vi "CheckI16_Range.vi"(8 "Step":i16, 11 "Current":i16) -> (3 "In Range Value":i16)   [LabVIEW 2016]
panel:
  # "Copyright (C) 2020 Edward S Allgeyer\n\nRedistribution and use in source and binary forms, with or without\nmodification, are permitted provided that the following conditions\nare met:\n\n1. Redistributions of source code must retain the above copyright\n   notice, this list of conditions and the following disclaimer.\n\n2. Redistributions in binary form must reproduce the above copyright\n   notice, this list of conditions and the following disclaimer in\n   the documentation and/or other materials provided with the\n   distribution.\n\n3. Neither the name of the copyright holder nor the names of its\n   contributors may be used to endorse or promote products derived\n   from this software without specific prior written permission.\n\nTHIS SOFTWARE IS PROVIDED BY THE COPYRIGHT HOLDERS AND CONTRIBUTORS\n\"AS IS\" AND ANY EXPRESS OR IMPLIED WARRANTIES, INCLUDING, BUT NOT\nLIMITED TO, THE IMPLIED WARRANTIES OF MERCHANTABILITY AND FITNESS\nFOR A PARTICULAR PURPOSE ARE DISCLAIMED. IN NO EVENT SHALL THE\nCOPYRIGHT HOLDER OR CONTRIBUTORS BE LIABLE FOR ANY DIRECT, INDIRECT,\nINCIDENTAL, SPECIAL, EXEMPLARY, OR CONSEQUENTIAL DAMAGES (INCLUDING,\nBUT NOT LIMITED TO, PROCUREMENT OF SUBSTITUTE GOODS OR SERVICES;\nLOSS OF USE, DATA, OR PROFITS; OR BUSINESS INTERRUPTION) HOWEVER\nCAUSED AND ON ANY THEORY OF LIABILITY, WHETHER IN CONTRACT, STRICT\nLIABILITY, OR TORT (INCLUDING NEGLIGENCE OR OTHERWISE) ARISING IN\nANY WAY OUT OF THE USE OF THIS SOFTWARE, EVEN IF ADVISED OF THE\nPOSSIBILITY OF SUCH DAMAGE."
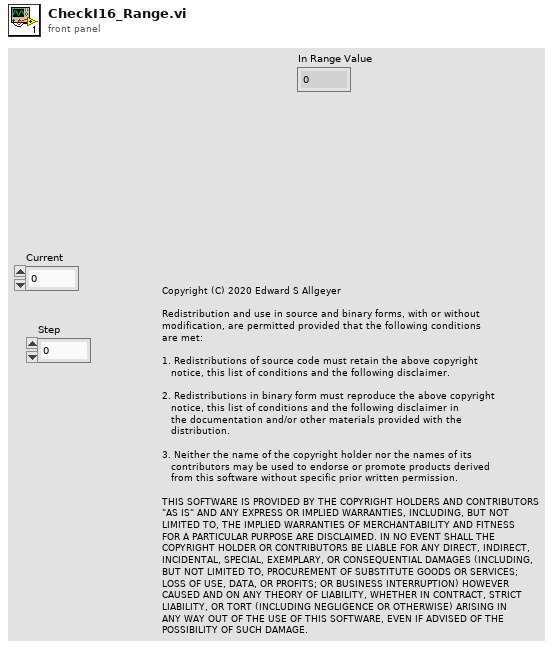
[diagram p1: front panel]
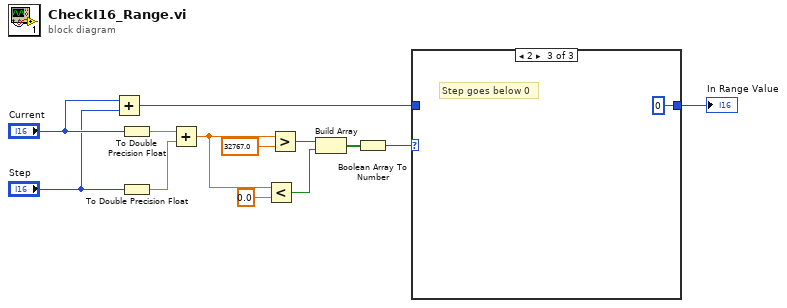
[diagram p0: block diagram]
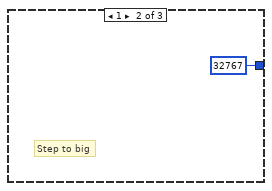
[diagram p3: hidden frame]
diagram:
  n1 = Add(x="Current", y="Step") -> (x+y=w2:i16)
  n2 = To Double Precision Float(number="Current") -> (double precision float=w13:dbl)
  n3 = To Double Precision Float(number="Step") -> (double precision float=w12:dbl)
  n4 = Add(x=w13, y=w12) -> (x+y=w10:dbl)
  n5 = Less?(x=w10, y=0.0) -> (x < y?=w7:bool)
  n6 = Greater?(x=w10, y=32767.0) -> (0:w8:bool)
  n7 = Build Array(w8, w7) -> (w6:bool[])
  n8 = Boolean Array To Number(Boolean array=w6) -> (number=w5:u32)
  n9 = case shown="2" w5 {
    tunnel: w2 -> [w14 _ _]
    tunnel: [w14 i16 32767 i16 0] -> w1
    frame 0, Default {
      # "In range"
    }
    frame 1 {
      # "Step to big"
    }
    frame 2 {
      # "Step goes below 0"
    }
  }
  "In Range Value" <- w1
